vi "Handle Depth Image.vi"(4 "queue in":refnum<queue>, 5 "Event Data":cluster{"sender":refnum<k24>, "e":refnum<k24>}, 6 "Control Ref":refnum<k24>, 7 "Event Common Data":T1) -> ()   [LabVIEW 2011]
uses:
  Microsoft.Kinect
  <vilib>/vision/Image Controls.llb/IMAQ Image.ctl
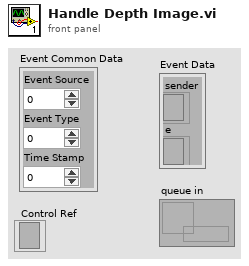
[diagram p1: front panel]
types:
  T1 = cluster{"Event Source":i32, "Event Type":u32, "Time Stamp":u32}
  T2 = typedef "Image Type" = u32
  T3 = typedef "IMAQ Image.ctl" = refnum<image>
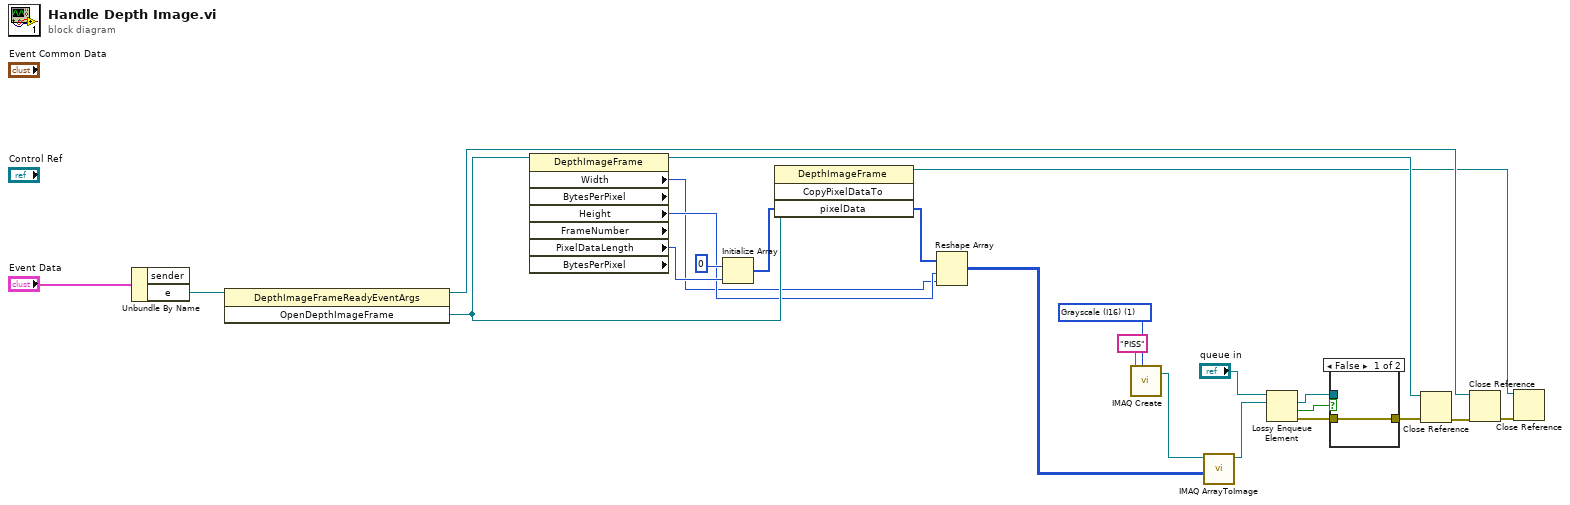
[diagram p0: block diagram]
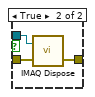
[diagram p2: hidden frame]
diagram:
  w18 = T2 1 items=["Grayscale (U8)", "Grayscale (I16)", "Grayscale (SGL)", "Complex (CSG)", "RGB (U32)", "HSL (U32)", "RGB (U64)", "Grayscale (U16)"] ("Image Type")
  n1 = Unbundle By Name("Event Data") -> ("e"=w24:refnum<k24>)  [unwired: 1 out]
  n2 = invoke class="DepthImageFrameReadyEventArgs" method="OpenDepthImageFrame"(reference=w24) -> (reference out=w12:refnum<k24>, "OpenDepthImageFrame"=w23:refnum<k24>)  [unwired: 2 in, 1 out]
  n3 = property on="Property Node" class="DepthImageFrame" props=["Width", "BytesPerPixel", "Height", "FrameNumber", "PixelDataLength", "BytesPerPixel"](reference=w23) -> (reference out=w14:refnum<k24>, "Width"=w2:i32, "Height"=w3:i32, "PixelDataLength"=w15:i32)  [unwired: 1 in, 4 out]
  n4 = Initialize Array(i16 0 ("element"), w15) -> (w22:i16[])
  n5 = invoke class="DepthImageFrame" method="CopyPixelDataTo"(reference=w23, "pixelData"=w22) -> (reference out=w4:refnum<k24>, "pixelData"=w16:i16[])  [unwired: 2 in, 2 out]
  n6 = Reshape Array(w16, w3, w2) -> (w1:i16[][])
  n7 = call "IMAQ Create"("Image Name"="PISS", "Image Type"=w18) -> ("New Image"=w19:T3)  [unwired: 3 in, 1 out]
  n8 = call "IMAQ ArrayToImage"("Image Pixels (I16)"=w1, "Image"=w19) -> ("Image Out"=w10:T3)  [unwired: 8 in, 1 out]
  n9 = Lossy Enqueue Element(queue="queue in", element=w10) -> (overflow element=w6:T3, overflow?=w8:bool, error out=w7:errorcluster)  [unwired: 1 in, 1 out]
  n10 = case shown="False" w8 {
    tunnel: w7 -> [w25 w28]
    tunnel: [w25 w27] -> w11
    tunnel: w6 -> [_ w26]
    frame False {
    }
    frame True {
      n11 = call "IMAQ Dispose"("Image"=w26, "error in (no error)"=w28) -> ("error out"=w27:errorcluster)  [unwired: 4 in]
    }
  }
  n12 = Close Reference(reference=w14, error in (no error)=w11) -> (error out=w13:errorcluster)
  n13 = Close Reference(reference=w12, error in (no error)=w13) -> (error out=w5:errorcluster)
  n14 = Close Reference(reference=w4, error in (no error)=w5) -> ()  [unwired: 1 out]
